vi "SRT-2014-Controls-Oxy.vi"() -> ()   [LabVIEW 2013]
uses:
  <vilib>/DAQmx/write.llb/DAQmx Write (Digital Bool 1Line 1Point).vi
  <vilib>/DAQmx/miscellaneous.llb/DAQmx Fill In Error Info.vi
panel:
  out "ESTES Ignition":bool
  out "O2 Ignite":bool
  in  "O2 Ignite":bool
  out "O2 Dropped":bool
  out "O2 Filling":bool
  in  "O2 Fill":bool
  out "NO2 Venting":bool
  out "NO2 Filling":bool
  in  "Emergency Stop":bool
  in  "Disconnected":bool
  in  "Done W/ NO2":bool
  in  "O2 Drop":bool
  in  "NO2 QD":bool
  in  "NO2 Vent":bool
  in  "NO2 Fill":bool
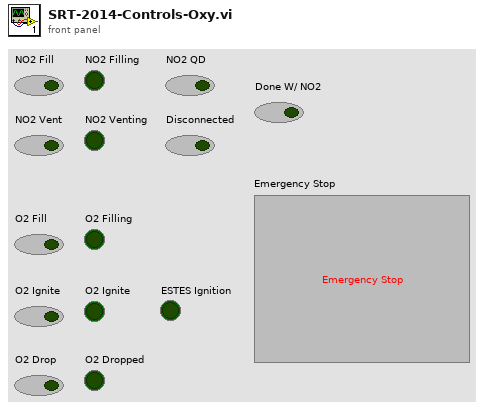
[diagram p1: front panel]
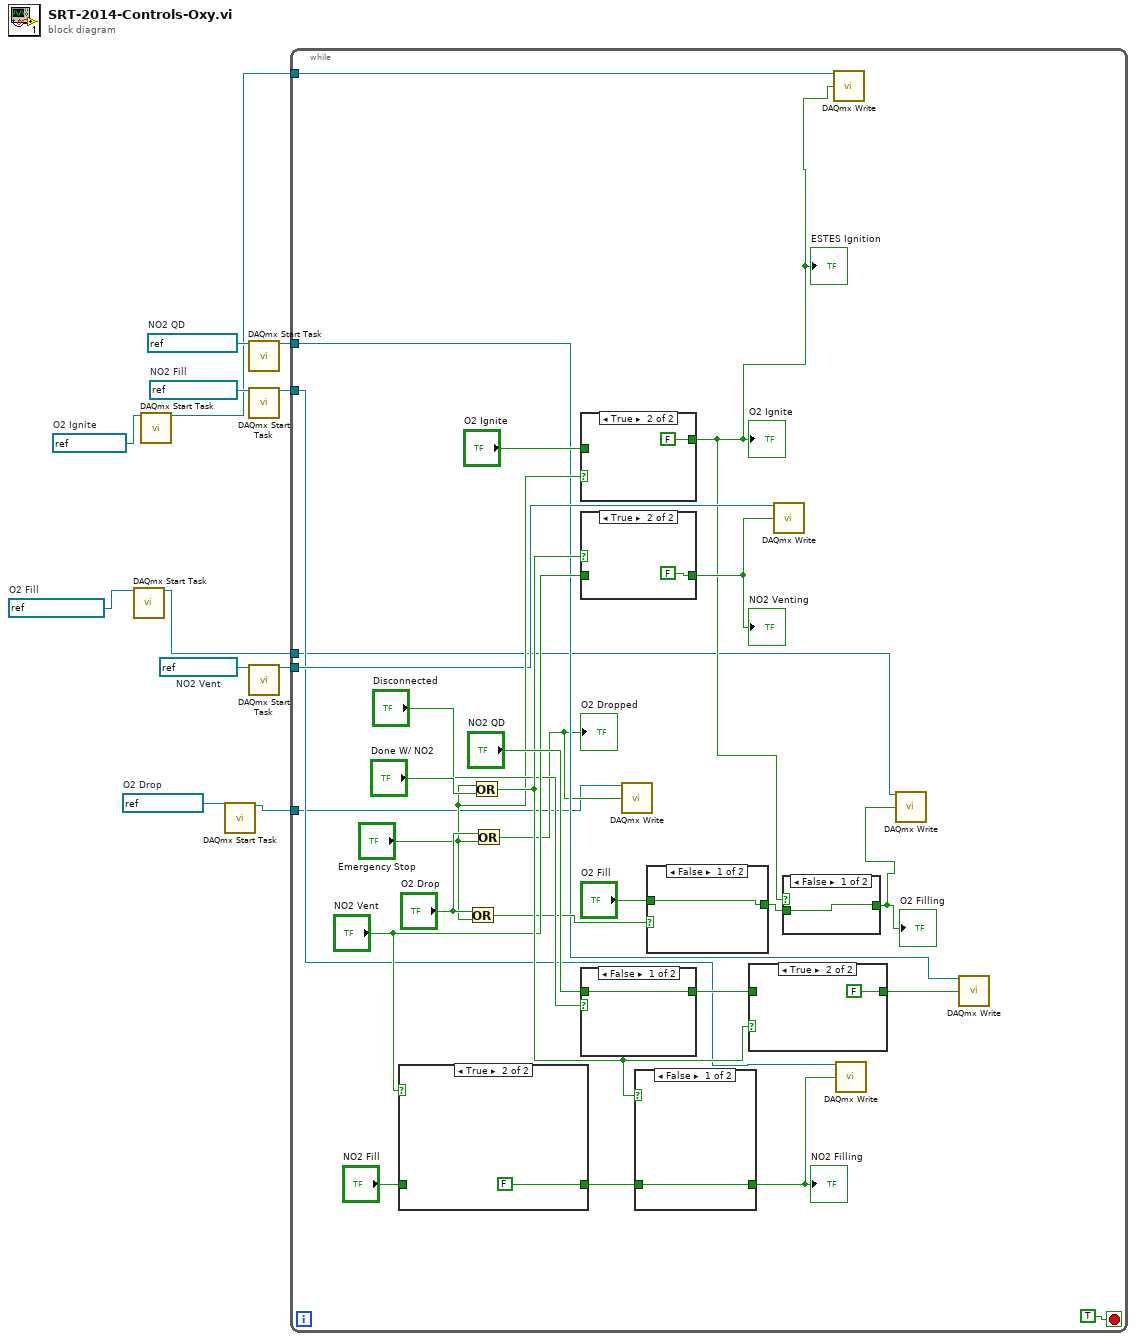
[diagram p0: block diagram]
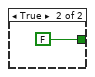
[diagram p2: hidden frame]
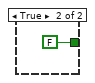
[diagram p4: hidden frame]
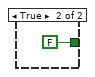
[diagram p6: hidden frame]
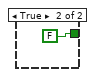
[diagram p8: hidden frame]
diagram:
  w10 = refnum<k21> "1_0"  # NO2 Fill
  w8 = refnum<k21> "1_2"  # NO2 QD
  w6 = refnum<k21> "2_3"  # O2 Ignite
  w5 = refnum<k21> "2_0"  # O2 Fill
  w4 = refnum<k21> "2_1"  # O2 Drop
  w12 = refnum<k21> "1_1"  # NO2 Vent
  n1 = call <vilib>:"DAQmx Start Task.vi"("task/channels in"=w5) -> ("task out"=w2:refnum<k21>)  [unwired: 13 in, 1 out]
  n2 = call <vilib>:"DAQmx Start Task.vi"("task/channels in"=w6) -> ("task out"=w3:refnum<k21>)  [unwired: 13 in, 1 out]
  n3 = call <vilib>:"DAQmx Start Task.vi"("task/channels in"=w4) -> ("task out"=w1:refnum<k21>)  [unwired: 13 in, 1 out]
  n4 = call <vilib>:"DAQmx Start Task.vi"("task/channels in"=w8) -> ("task out"=w7:refnum<k21>)  [unwired: 13 in, 1 out]
  n5 = call <vilib>:"DAQmx Start Task.vi"("task/channels in"=w10) -> ("task out"=w9:refnum<k21>)  [unwired: 13 in, 1 out]
  n6 = call <vilib>:"DAQmx Start Task.vi"("task/channels in"=w12) -> ("task out"=w11:refnum<k21>)  [unwired: 13 in, 1 out]
  n7 = while {
    tunnel: w11 -> [w25]
    tunnel: w9 -> [w23]
    tunnel: w7 -> [w21]
    tunnel: w3 -> [w18]
    tunnel: w2 -> [w16]
    tunnel: w1 -> [w13]
    stop <- TRUE stop-if-true
    n8 = case shown="True" "NO2 Vent" {
      tunnel: "NO2 Fill" -> [w54 _]
      tunnel: [w54 FALSE] -> w37
      frame False {
      }
      frame True {
      }
    }
    n9 = Or(x="O2 Drop", y="Emergency Stop") -> (x .or. y?=w29:bool)
    n10 = Or(x="Emergency Stop", y="Done W/ NO2") -> (x .or. y?=w34:bool)
    n11 = Or(x="O2 Drop", y="Emergency Stop") -> (x .or. y?=w14:bool)
    "O2 Dropped" <- w14
    n12 = case shown="True" "Emergency Stop" {
      tunnel: [w42 FALSE] -> w17
      tunnel: "O2 Ignite" -> [w42 _]
      frame False {
      }
      frame True {
      }
    }
    "O2 Ignite" <- w17
    "ESTES Ignition" <- w17
    n13 = case shown="True" w34 {
      tunnel: [w50 FALSE] -> w24
      tunnel: "NO2 Vent" -> [w50 _]
      frame False {
      }
      frame True {
      }
    }
    "NO2 Venting" <- w24
    n14 = case shown="False" "Disconnected" {
      tunnel: "NO2 QD" -> [w52 _]
      tunnel: [w52 FALSE] -> w36
      frame False {
      }
      frame True {
      }
    }
    n15 = call-poly <vilib>:"DAQmx Write.vi"("task/channels in"=w13, "data"=w14) -> ()  [unwired: 11 in, 3 out]
    n16 = case shown="False" w34 {
      tunnel: w37 -> [w48 _]
      tunnel: [w48 FALSE] -> w22
      frame False {
      }
      frame True {
      }
    }
    "NO2 Filling" <- w22
    n17 = case shown="False" w29 {
      tunnel: [w44 FALSE] -> w19
      tunnel: "O2 Fill" -> [w44 _]
      frame False {
      }
      frame True {
      }
    }
    n18 = case shown="True" w34 {
      tunnel: w36 -> [w46 _]
      tunnel: [w46 FALSE] -> w20
      frame False {
      }
      frame True {
      }
    }
    n19 = call-poly <vilib>:"DAQmx Write.vi"("task/channels in"=w25, "data"=w24) -> ()  [unwired: 11 in, 3 out]
    n20 = case shown="False" w17 {
      tunnel: [w40 FALSE] -> w15
      tunnel: w19 -> [w40 _]
      frame False {
      }
      frame True {
      }
    }
    "O2 Filling" <- w15
    n21 = call-poly <vilib>:"DAQmx Write.vi"("task/channels in"=w18, "data"=w17) -> ()  [unwired: 11 in, 3 out]
    n22 = call-poly <vilib>:"DAQmx Write.vi"("task/channels in"=w23, "data"=w22) -> ()  [unwired: 11 in, 3 out]
    n23 = call-poly <vilib>:"DAQmx Write.vi"("task/channels in"=w16, "data"=w15) -> ()  [unwired: 11 in, 3 out]
    n24 = call-poly <vilib>:"DAQmx Write.vi"("task/channels in"=w21, "data"=w20) -> ()  [unwired: 11 in, 3 out]
  }
